vi "JSON_Patcher.vi"(7 "Küldési Mód":string(combo)="PATCH", 10 "JSON utvonal":string, 11 "JSON_string":string) -> (2 "standard output":string)   [LabVIEW 2015]
uses:
  <vilib>/Platform/system.llb/System Exec.vi
panel:
  out "concatenated string":string
  out "CMD string":string
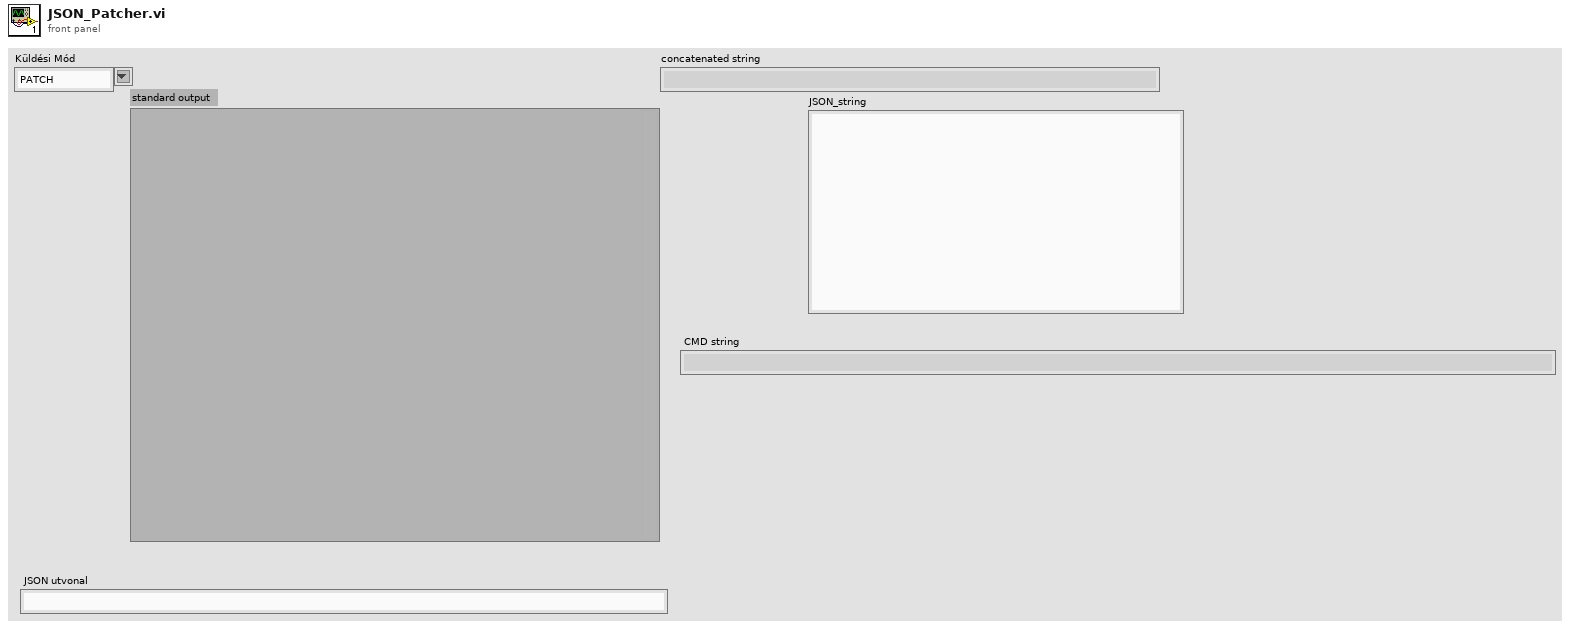
[diagram p1: front panel]
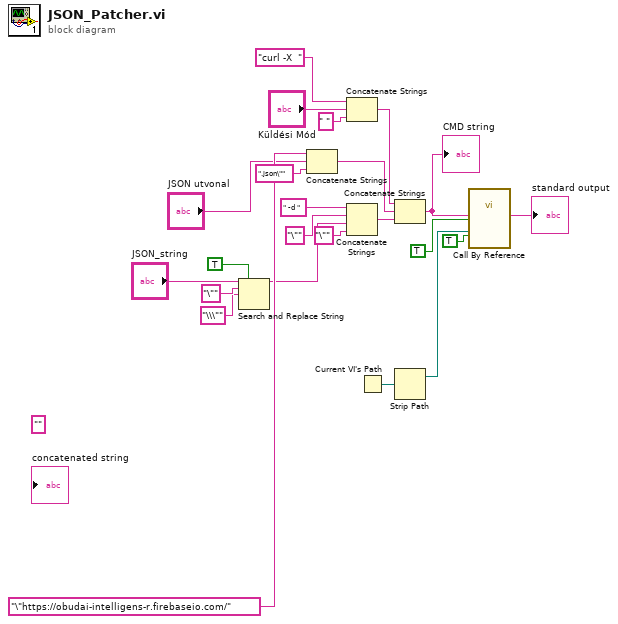
[diagram p0: block diagram]
diagram:
  (unwired) "" ("string")
  n1 = Search and Replace String(replace all?=TRUE ("replace all? (F)"), input string="JSON_string", search string="\"", replace string="\\\"" ("replace string (\"\")")) -> (result string=w1:string)  [unwired: 4 in, 3 out]
  n2 = Concatenate Strings("\"https://obudai-intelligens-r.firebaseio.com/" ("url"), "JSON utvonal", ".json\"" ("string")) -> (w8:string)
  n3 = Concatenate Strings("curl -X  " ("string"), "Küldési Mód", " " ("string")) -> (w11:string)
  n4 = Concatenate Strings(" -d " ("string"), "\"" ("string"), w1, "\"" ("string")) -> (w7:string)
  n5 = Current VI's Path() -> (path=w21:path)
  n6 = Concatenate Strings(w11, w8, w7) -> (w16:string)
  "CMD string" <- w16
  n7 = Strip Path(path=w21) -> (stripped path=w20:path)  [unwired: 1 out]
  n8 = call-by-ref "?"("run minimized? (F)"=TRUE, "wait until completion? (T)"=TRUE, "working directory"=w20, "command line"=w16) -> ("standard output"=→"standard output":string)  [unwired: 6 in, 5 out]
